vi "DMC Tools.vi"() -> ()   [LabVIEW 2021]
panel:
  in  "Open Button":bool
  in  "New Folder Button":bool
  in  "Copy Button":bool
  in  "Graph Button":bool
  in  "Chart Button":bool
  in  "Home Button":bool
  in  "Control Button":bool
  in  "Date Time Button":bool
  in  "Clock Button":bool
  in  "Alarm Button":bool
  in  "Add Alarm Button":bool
  in  "Search Button":bool
  in  "Power Button":bool
  in  "Reset Button":bool
  in  "Refresh Button":bool
  in  "Close Button":bool
  in  "OK Button":bool
  in  "Delete Button":bool
  in  "Edit Button":bool
  in  "Tools Button":bool
  in  "Settings Button":bool
  in  "Save Button":bool
  in  "Report Button":bool
  in  "View Button":bool
  in  "Stop Button":bool
  in  "Pause Button":bool
  in  "Start Button":bool
  in  "Upload Button":bool
  in  "Download Button":bool
  in  "Unlock Button":bool
  in  "Lock Button":bool
  in  "Forward Button":bool
  in  "Back Button":bool
  in  "Down Button":bool
  in  "Up Button":bool
  in  "Cancel Button":bool
  in  "Help Button":bool
  in  "Information Button":bool
  in  "Warning Button":bool
  in  "Remove Button":bool
  in  "Add Button":bool
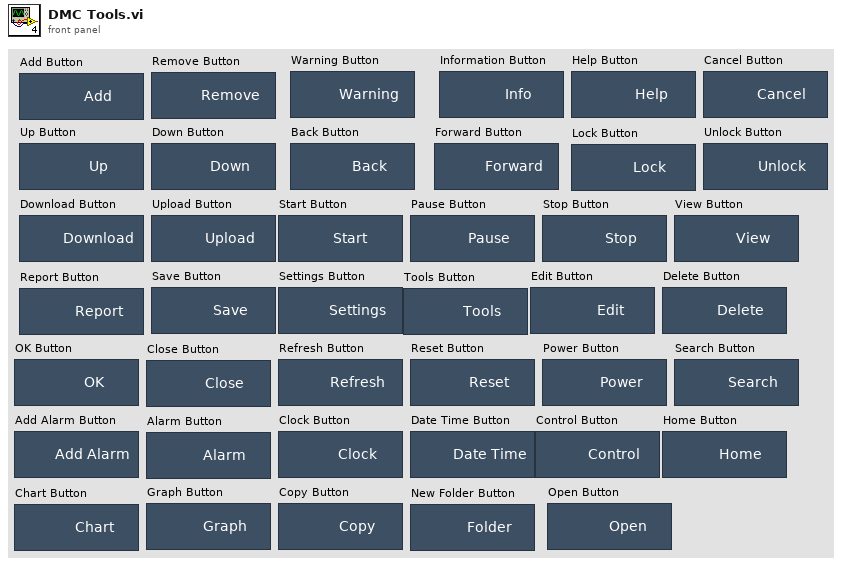
[diagram p1: front panel]
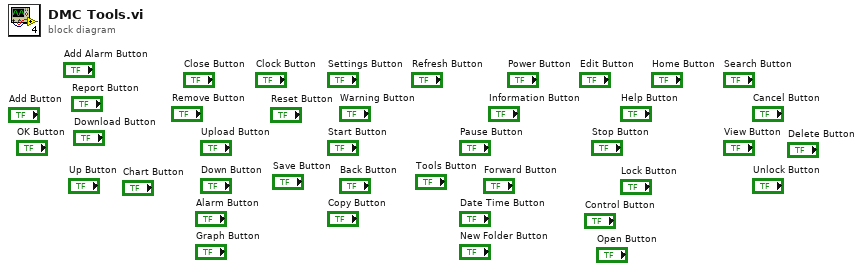
[diagram p0: block diagram]
diagram:
